vi "read data.vi"(8 "error in (no error)":errorcluster, 11 "NI-9237 in":refnum<class "NI-9237.lvclass">) -> (0 "error out":errorcluster, 3 "NI-9237 out":refnum<class "NI-9237.lvclass">)   [LabVIEW 2025, in "Wheatstone Bridge.lvlib" / "NI-9237.lvclass"]
uses:
  NI-9237.lvclass
  NI-9237.lvclass/NI-9237.ctl
  <vilib>/DAQmx/read.llb/DAQmx Read (Analog DBL 1Chan 1Samp).vi
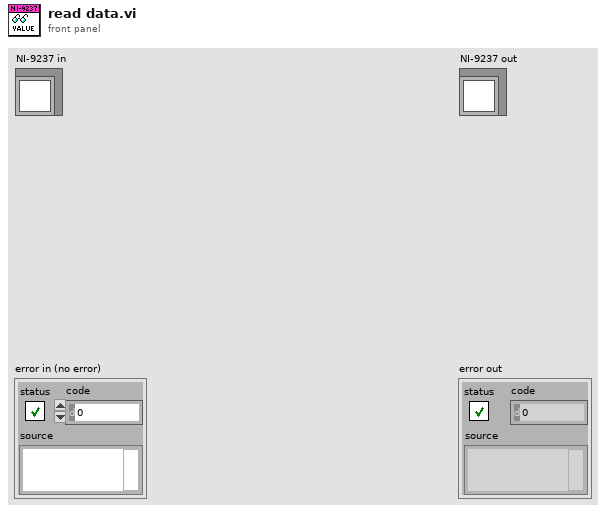
[diagram p1: front panel]
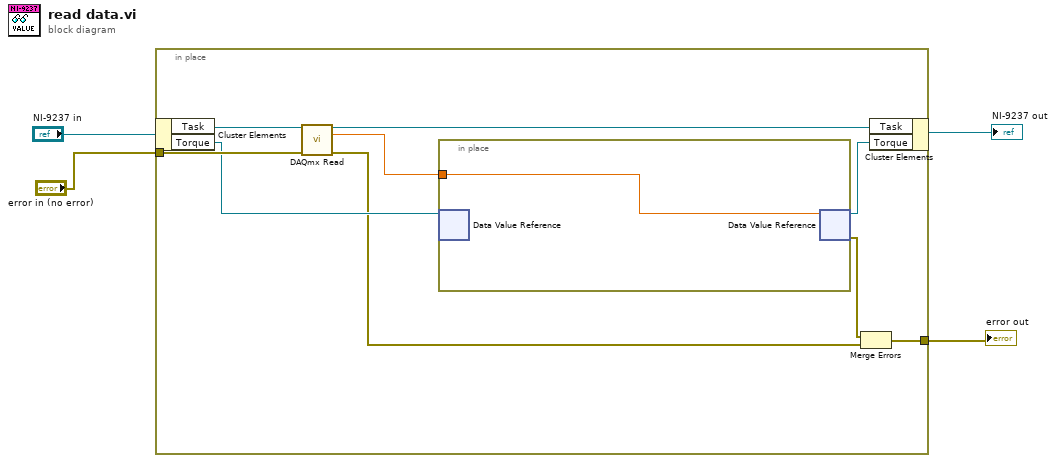
[diagram p0: block diagram]
diagram:
  n1 = in-place {
    in-place-border: "error in (no error)" -> [w11]
    in-place-border: [w7] -> w2
    n2 = in-place-cluster #1("NI-9237 in") -> ("Task"=w13:refnum<k21>, "Torque"=w10:refnum<data-value>)
    n3 = call-poly <vilib>:"DAQmx Read.vi"("task/channels in"=w13, "error in"=w11) -> ("task out"=w12:refnum<k21>, "data"=w9:dbl, "error out"=w5:errorcluster)  [unwired: 11 in]
    n4 = in-place {
      in-place-border: w9 -> [w14]
      n5 = in-place-dvr #2(w10) -> ()  [unwired: 2 out]
      n6 = in-place-dvr #2(w14) -> (w8:refnum<data-value>, w6:errorcluster)
    }
    n7 = Merge Errors(w6, w5) -> (w7:errorcluster)
    n8 = in-place-cluster #1("Task"=w12, "Torque"=w8) -> (→"NI-9237 out":refnum<class "NI-9237.lvclass">)
  }
  "error out" <- w2
